vi "Robot_Targeting_adjustment.vi"() -> ()   [LabVIEW 2018]
uses:
  <vilib>/Rock Robotics/Network Tables/NT Read Number.vi
  <vilib>/addons/control/pid/pid.llb/PID (DBL).vi
  <vilib>/addons/control/pid/NI_PID_pid.lvlib
panel:
  in  "Tape Strafe":T1={"proportional gain (Kc)"=0.035, "integral time (Ti, min)"=0.0, "derivative time (Td, min)"=0.0018} {"derivative time (Td, min)" format="%.3f"; "integral time (Ti, min)" format="%.3f"; "proportional gain (Kc)" format="%.3f"}
  in  "Tape Range":cluster{"output high":dbl, "output low":dbl}={"output high"=0.7, "output low"=-0.7} {"output low" format="%.2f"; "output high" format="%.2f"}
  in  "Ball Range":cluster{"output high":dbl, "output low":dbl}={"output high"=0.7, "output low"=-0.7} {"output low" format="%.2f"; "output high" format="%.2f"}
  in  "Ball Rotate":T1={"proportional gain (Kc)"=0.035, "integral time (Ti, min)"=0.0, "derivative time (Td, min)"=0.0018} {"derivative time (Td, min)" format="%.3f"; "integral time (Ti, min)" format="%.3f"; "proportional gain (Kc)" format="%.3f"}
  # ".7\n-.7"
  # "1\n-1"
  # ".5\n-.5"
  # "Rotation"
  # "Strafe"
  # "Forward back"
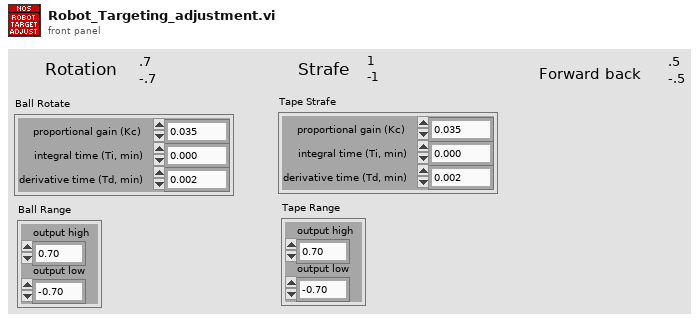
[diagram p1: front panel]
types:
  T1 = cluster{"proportional gain (Kc)":dbl, "integral time (Ti, min)":dbl, "derivative time (Td, min)":dbl}
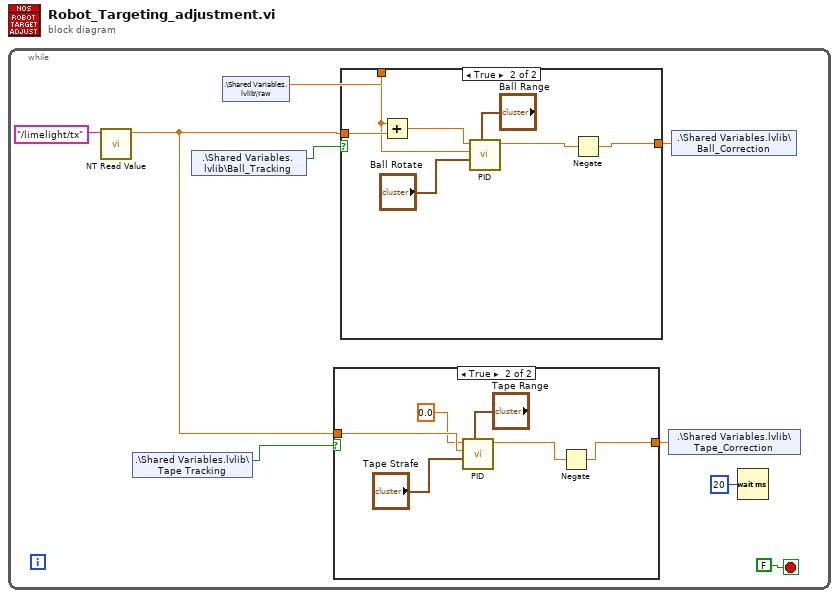
[diagram p0: block diagram]
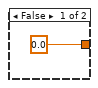
[diagram p2: hidden frame]
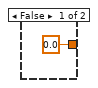
[diagram p3: hidden frame]
diagram:
  n1 = while {
    stop <- FALSE stop-if-true
    n2 = call-poly <vilib>:"NT Read Value.vi"("Name"="/limelight/tx") -> ("Numeric"=w5:dbl)  [unwired: 9 in, 1 out]
    n3 = shared-variable ".\\Shared Variables.lvlib\\Tape Tracking"() -> (w4:bool)  [unwired: 1 in, 1 out]
    n4 = shared-variable ".\\Shared Variables.lvlib\\Ball_Tracking"() -> (w8:bool)  [unwired: 1 in, 1 out]
    n5 = shared-variable ".\\Shared Variables.lvlib\\Yaw"() -> (w7:dbl)  [unwired: 1 in, 1 out]
    n6 = case shown="True" w4 {
      tunnel: w5 -> [_ w14]
      tunnel: [0.0 ("output") w11] -> w2
      frame False {
      }
      frame True {
        n7 = call-poly <vilib>:"PID.vi"("output range"="Tape Range", "PID gains"="Tape Strafe", "process variable"=w14, "setpoint"=0.0) -> ("output"=w12:dbl)  [unwired: 6 in, 1 out]
        n8 = Negate(x=w12) -> (-x=w11:dbl)
      }
    }
    n9 = case shown="True" w8 {
      tunnel: w7 -> [_ w22]
      tunnel: w5 -> [_ w24]
      tunnel: [0.0 ("output") w18] -> w3
      frame False {
      }
      frame True {
        n10 = Add(x=w22, y=w24) -> (x+y=w23:dbl)
        n11 = call-poly <vilib>:"PID.vi"("output range"="Ball Range", "PID gains"="Ball Rotate", "process variable"=w22, "setpoint"=w23) -> ("output"=w19:dbl)  [unwired: 6 in, 1 out]
        n12 = Negate(x=w19) -> (-x=w18:dbl)
      }
    }
    n13 = shared-variable ".\\Shared Variables.lvlib\\Tape_Correction"(w2) -> ()  [unwired: 1 in, 1 out]
    n14 = shared-variable ".\\Shared Variables.lvlib\\Ball_Correction"(w3) -> ()  [unwired: 1 in, 1 out]
    n15 = Wait (ms)(milliseconds to wait=u32 20) -> ()  [unwired: 1 out]
  }
